vi "문자열저장.vi"() -> ()   [LabVIEW 2014]
uses:
  <vilib>/Analysis/NI_AALBase.lvlib
panel:
  out "스프레드시트 문자열":string
  out "테이블 컨트롤":string[][](table)
  out "웨이브폼 그래프":dbl[][](graph)
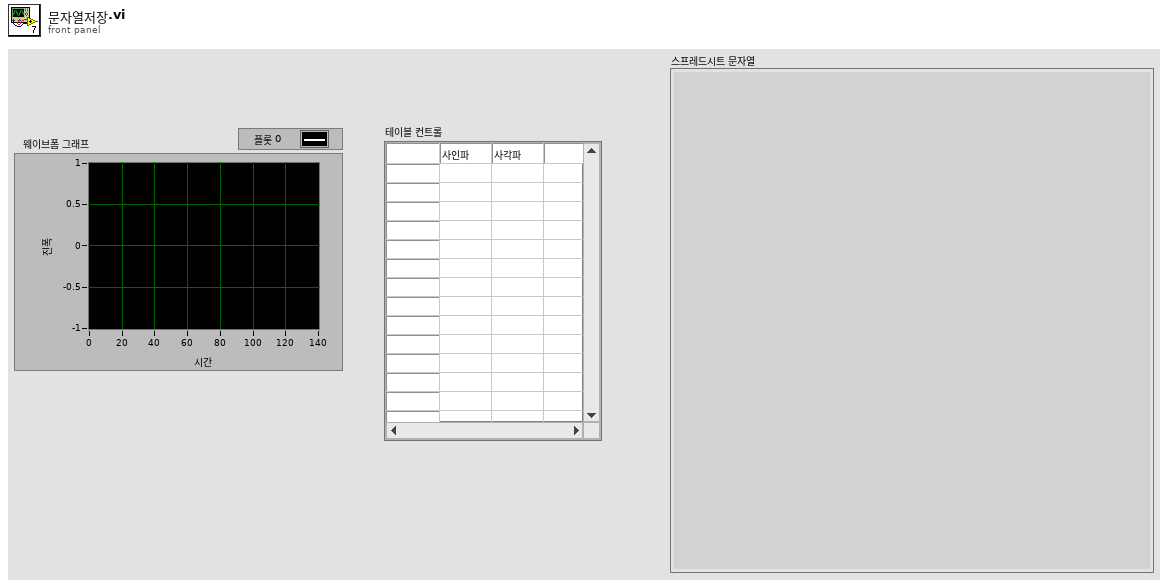
[diagram p1: front panel]
types:
  T1 = enum16{"open", "replace", "create", "open or create", "replace or create", "replace or create with confirmation"}
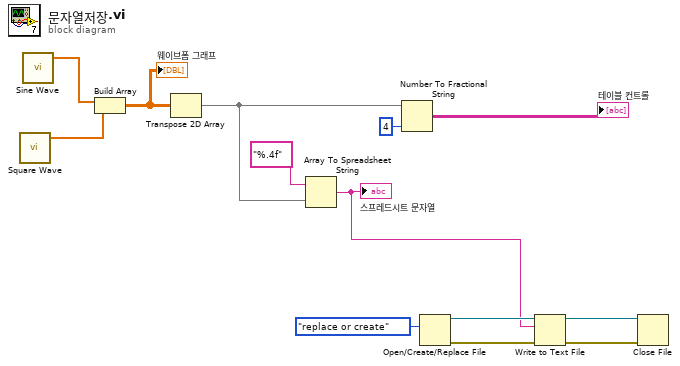
[diagram p0: block diagram]
diagram:
  n1 = call <vilib>:"Square Wave.vi"() -> ("square wave"=w11:dbl[])  [unwired: 6 in, 2 out]
  n2 = call <vilib>:"Sine Wave.vi"() -> ("sine wave"=w12:dbl[])  [unwired: 5 in, 2 out]
  n3 = Build Array(w12, w11) -> (w10:dbl[][])
  "웨이브폼 그래프" <- w10
  n4 = Transpose 2D Array(2D array=w10) -> (transposed array=w8:dbl[][])
  n5 = Array To Spreadsheet String(array=w8, 3:"%.4f" ("포맷 문자열")) -> (spreadsheet string=w1:string)  [unwired: 1 in]
  "스프레드시트 문자열" <- w1
  n6 = Number To Fractional String(number=w8, precision (6)=i16 4 ("정밀도(6)")) -> (F-format string=→"테이블 컨트롤":string[][])  [unwired: 2 in]
  n7 = Open/Create/Replace File(operation (0:open)=T1."replace or create" ("동작(0:open)")) -> (refnum out=w6:refnum<file>, error out=w4:errorcluster)  [unwired: 5 in, 1 out]
  n8 = Write to Text File(file (use dialog)=w6, text=w1, error in=w4) -> (refnum out=w5:refnum<file>, error out=w3:errorcluster)  [unwired: 1 in, 1 out]
  n9 = Close File(refnum=w5, error in=w3) -> ()  [unwired: 2 out]
